vi "Actor Core.vi"(8 "error in":errorcluster, 11 "Measure Object in":refnum<class "Measure Object.lvclass">) -> (0 "error out":errorcluster, 3 "Actor out":refnum<class "Actor.lvclass">)   [LabVIEW 2015, in "Measure Object.lvclass"]
doc: "(<B>Filename</B>: Actor Framework.lvlib:Actor.lvclass:Actor Core.vi)\n\nReceives messages to the actor, reacts to them, and initiates any error handling that may shut the actor down.\n\nDescendant classes may override this VI to append parallel tasks for the actor to complete while it handles messages. Overrides use the Call Parent Method node."
uses:
  Measure Object.lvclass
  <vilib>/ActorFramework/Actor/Actor.lvclass
  <vilib>/ActorFramework/Actor/Actor.lvclass/Actor.ctl
  <vilib>/ActorFramework/Message Enqueuer/Message Enqueuer.lvclass/Message Enqueuer.ctl
  Measure Object.lvclass/Measure Object.ctl
  Measure Object Messages/Open Item Msg/Open Item Msg.lvclass/Open Item Msg.ctl
  <vilib>/ActorFramework/Message Enqueuer/Init from Existing Queue.vi
  <vilib>/ActorFramework/Message Enqueuer/Enqueue.vi
  <vilib>/ActorFramework/Message Priority Queue/Priority Enqueue.vi
  <vilib>/ActorFramework/Message Enqueuer/Message Enqueuer.lvclass
  Measure Object Messages/Open Item Msg/Open Item Msg.lvclass
panel:
  in  "No UI has been defined for this object":bool
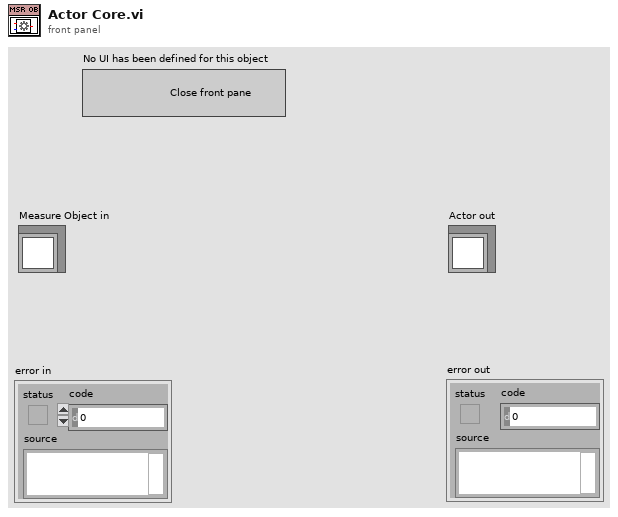
[diagram p1: front panel]
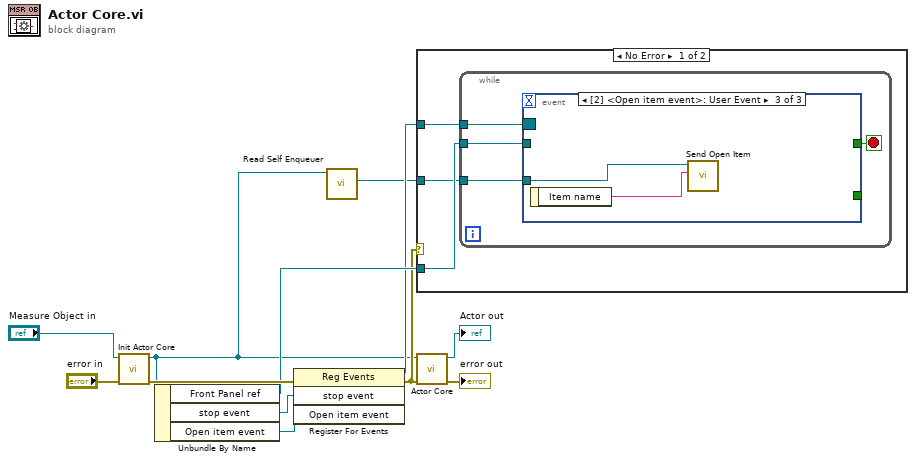
[diagram p0: block diagram]
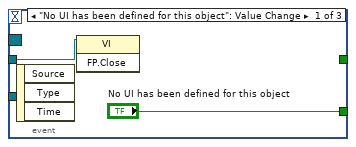
[diagram p2: hidden frame]
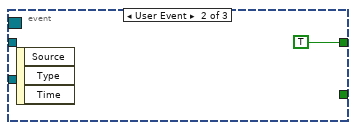
[diagram p3: hidden frame]
diagram:
  n1 = call-dynamic "Init Actor Core.vi"("error in (no error)"="error in", "Measure Object in"="Measure Object in") -> ("error out"=w8:errorcluster, "Measure Object out"=w2:refnum<class "Measure Object.lvclass">)  [unwired: 8 in]
  n2 = Unbundle By Name(w2) -> ("Front Panel ref"=w5:refnum<vi>, "stop event"=w7:refnum<user-event>, "Open item event"=w6:refnum<user-event>)
  n3 = register-events(error in=w8, w7, w6) -> (reference out=w4:refnum<event-registration>, error out=w3:errorcluster)  [unwired: 1 in]
  n4 = call <vilib>:"Read Self Enqueuer.vi"("Actor"=w2) -> ("Self Enqueuer"=w1:refnum<class "Message Enqueuer.lvclass">)  [unwired: 10 in]
  n5 = case shown="No Error" w3 {
    tunnel: w5 -> [w15 _]
    tunnel: w4 -> [w14 _]
    tunnel: w1 -> [w13 _]
    frame No Error {
      n6 = while {
        tunnel: w15 -> [w19]
        tunnel: w14 -> [w18]
        tunnel: w13 -> [w16]
        stop <- w17 stop-if-true
        n7 = event shown="[2] <Open item event>: User Event" {
          selector: w18 -> [_ _ _]
          dyn-events: _ -> [_ _ _]
          timeout: _ -> [_ _ _]
          tunnel: w19 -> [w21 _ _]
          tunnel: ["No UI has been defined for this object" _ _] -> _
          tunnel: [_ TRUE _] -> w17
          tunnel: w16 -> [_ _ w24]
          event "No UI has been defined for this object": Value Change {
            n8 = event-data() -> ()  [unwired: 1 in, 3 out]
            n9 = invoke class="VI" method="FP.Close"(reference=w21) -> ()  [unwired: 2 in, 3 out]
          }
          event User Event {
            n10 = event-data() -> ()  [unwired: 1 in, 3 out]
          }
          event User Event {
            n11 = event-data() -> ("Item name"=w23:string)  [unwired: 1 in]
            n12 = call "Send Open Item.vi"("Item name"=w23, "Message Enqueuer"=w24) -> ()  [unwired: 8 in, 2 out]
          }
        }
      }
    }
    frame Error {
    }
  }
  n13 = call-parent "Actor Core.vi"("error in"=w3, "Actor in"=w2) -> ("error out"=→"error out":errorcluster, "Actor out"=→"Actor out":refnum<class "Actor.lvclass">)  [unwired: 8 in]
